vi "Initialize.vi"(8 "error IO":errorcluster, 10 "Software version":string="v1.14.0", 11 "Channel.lvclass":refnum<class "SPARC4_Channel.lvclass">) -> (0 "error IO 2":errorcluster, 3 "Channel.lvclass 2":refnum<class "SPARC4_Channel.lvclass">)   [LabVIEW 2018, in "SPARC4_Channel.lvclass"]
doc: "Initialize ACS"
uses:
  SPARC4_Channel.lvclass
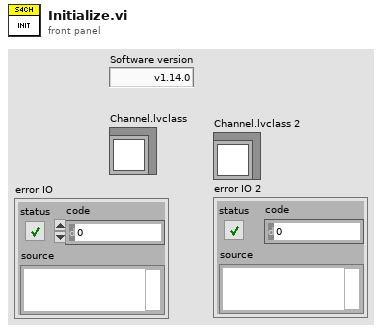
[diagram p1: front panel]
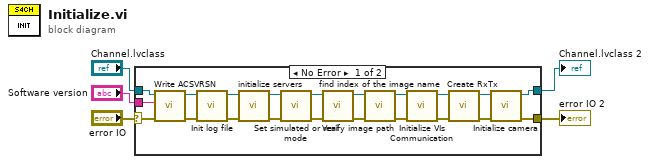
[diagram p0: block diagram]
diagram:
  n1 = case shown="No Error" "error IO" {
    selector: "error IO" -> [w23 w28]
    tunnel: [w18 w28] -> w2
    tunnel: [w19 w27] -> w3
    tunnel: "Channel.lvclass" -> [w15 w27]
    tunnel: "Software version" -> [w20 _]
    frame No Error {
      n2 = call "Write ACSVRSN.vi"("error in (no error)"=w23, "ACSVRSN"=w20, "Channel in"=w15) -> ("error out"=w8:errorcluster, "Channel out"=w11:refnum<class "SPARC4_Channel.lvclass">)  [unwired: 7 in]
      n3 = call "Init log file.vi"("error in (no error)"=w8, "Channel in"=w11) -> ("error out"=w9:errorcluster, "Channel out"=w10:refnum<class "SPARC4_Channel.lvclass">)  [unwired: 8 in]
      n4 = call "initialize servers.vi"("error in (no error)"=w9, "Channel in"=w10) -> ("error out"=w12:errorcluster, "Channel out"=w13:refnum<class "SPARC4_Channel.lvclass">)  [unwired: 8 in]
      n5 = call "Set simulated or real mode.vi"("error in (no error)"=w12, "Channel in"=w13) -> ("error out"=w21:errorcluster, "Channel out"=w22:refnum<class "SPARC4_Channel.lvclass">)  [unwired: 8 in]
      n6 = call "Verify image path.vi"("error in (no error)"=w21, "Channel in"=w22) -> ("error out"=w6:errorcluster, "Channel out"=w7:refnum<class "SPARC4_Channel.lvclass">)  [unwired: 8 in]
      n7 = call "find index of the image name.vi"("error in (no error)"=w6, "Channel in"=w7) -> ("error out"=w24:errorcluster, "Channel out"=w14:refnum<class "SPARC4_Channel.lvclass">)  [unwired: 8 in]
      n8 = call "Initialize VIs Communication.vi"("error in (no error)"=w24, "Channel in"=w14) -> ("error out"=w25:errorcluster, "Channel out"=w26:refnum<class "SPARC4_Channel.lvclass">)  [unwired: 8 in]
      n9 = call "Create RxTx.vi"("error in (no error)"=w25, "Channel in"=w26) -> ("error out"=w16:errorcluster, "Channel out"=w17:refnum<class "SPARC4_Channel.lvclass">)  [unwired: 8 in]
      n10 = call "Initialize camera.vi"("error in (no error)"=w16, "Channel in"=w17) -> ("error out"=w18:errorcluster, "Channel out"=w19:refnum<class "SPARC4_Channel.lvclass">)  [unwired: 8 in]
    }
    frame Error {
    }
  }
  "Channel.lvclass 2" <- w3
  "error IO 2" <- w2
